vi "plotToString.vi"(8 "Precision2":string, 9 "Precision1":string, 10 "Column2":dbl[](array[numeric]), 11 "Column1":dbl[](array[numeric])) -> (2 "nLoops":i32, 3 "plotString":string)   [LabVIEW 2013]
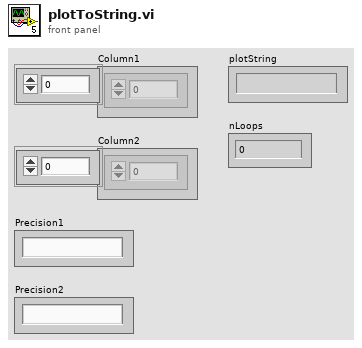
[diagram p1: front panel]
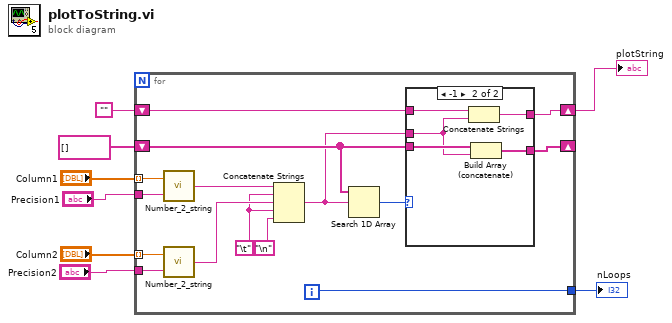
[diagram p0: block diagram]
diagram:
  n1 = for {
    tunnel: "Column1" -> [w23] mode=indexing
    shift-right: [w18] -> w1
    shift-left: "" -> [w19]
    tunnel: "Column2" -> [w11] mode=indexing
    shift-right: [w17] -> _
    shift-left: string[] [] -> [w16]
    tunnel: "Precision1" -> [w13]
    tunnel: "Precision2" -> [w12]
    tunnel: [w9] -> w8
    i -> [w9]
    w20 = "\t"
    n2 = call "Number_2_string.vi"("precision"=w13, "number"=w23) -> ("String"=w22:string)
    n3 = call "Number_2_string.vi"("precision"=w12, "number"=w11) -> ("String"=w21:string)
    n4 = Concatenate Strings(w22, w20, w21, w20, "\n") -> (w15:string)
    n5 = Search 1D Array(1D array=w16, element=w15) -> (index of element=w14:i32)  [unwired: 1 in]
    n6 = case shown="-1" w14 {
      tunnel: w19 -> [w25 w30]
      tunnel: [w25 w29] -> w18
      tunnel: w15 -> [_ w26]
      tunnel: w16 -> [w24 w28]
      tunnel: [w24 w27] -> w17
      frame 0, Default {
      }
      frame -1 {
        n7 = Concatenate Strings(w30, w26) -> (w29:string)
        n8 = Build Array (concatenate)(w28, w26) -> (w27:string[])
      }
    }
  }
  "nLoops" <- w8
  "plotString" <- w1
